vi "GetLedStates.vi"(8 "error in (no error)":errorcluster, 10 "ChainNumber":u8, 11 "ControlState in":T1 {"ChainMask" format="0x%02x"}) -> (0 "error out":errorcluster, 2 "LED Colors":u32[](array[colorbox]), 3 "ControlState out":T1 {"ChainMask" format="0x%02x"})   [LabVIEW 2023, in "ArduinoSerialBling.lvlib"]
uses:
  ArduinoSerialBling.lvlib
  ControlState.ctl
  ChainState.ctl
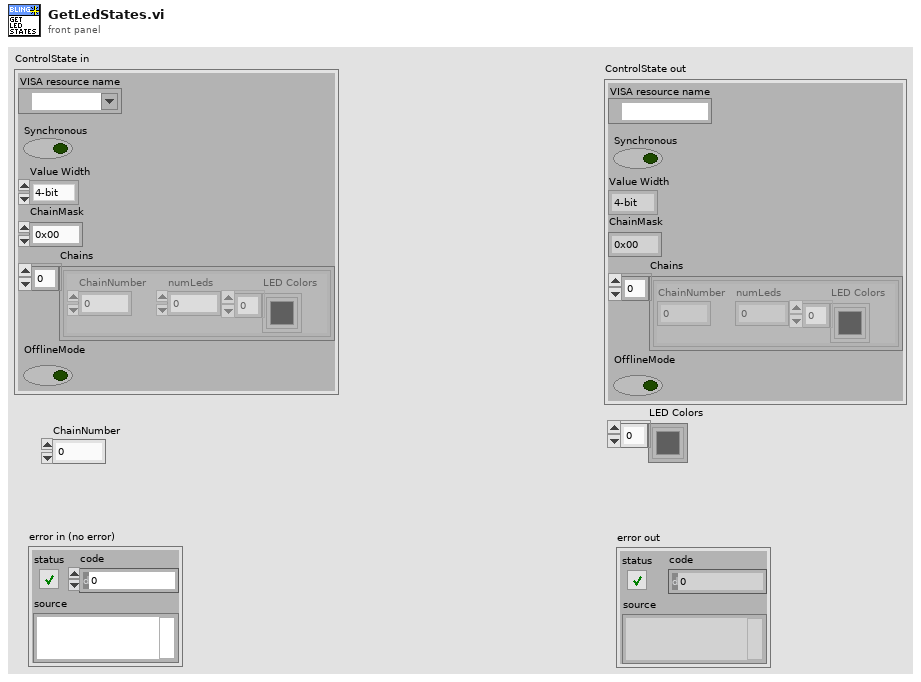
[diagram p1: front panel]
types:
  T1 = typedef "ArduinoSerialBling.lvlib/ControlState.ctl" = cluster{"VISA resource name":refnum<visa-resource-name>, "Synchronous":bool, "Value Width":enum16{"4-bit", "8-bit"}, "ChainMask":u8, "Chains":T2[], "OfflineMode":bool}
  T2 = typedef "ArduinoSerialBling.lvlib/ChainState.ctl" = cluster{"ChainNumber":u8, "numLeds":u8, "LED Colors":u32[]}
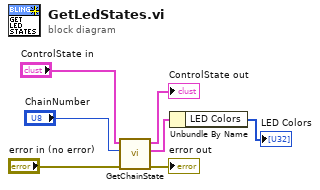
[diagram p0: block diagram]
diagram:
  n1 = call "GetChainState.vi"("error in (no error)"="error in (no error)", "ChainNumber"="ChainNumber", "ControlState in"="ControlState in") -> ("error out"=→"error out":errorcluster, "ChainState"=w2:T2, "ControlState out"=→"ControlState out":T1)  [unwired: 5 in, 1 out]
  n2 = Unbundle By Name(w2) -> ("LED Colors"=→"LED Colors":u32[])
